vi "mupExpr Demo1.vi"() -> ()   [LabVIEW 2015]
uses:
  mupExpr/mupExpr.lvclass/mupExpr.ctl
  mupExpr/SetVarVal.vi
  mupLib/mupEval.vi
  mupLib/mupSetVarValue.vi
  mupLib/mupCheckError.vi
  mupLib/mupLibPath.vi
  <vilib>/Utility/error.llb/Error Cluster From Error Code.vi
  mupExpr/mupExpr.lvclass
panel:
  in  "Constants":cluster{"name":string, "value":dbl}[](array[cluster])=[{"name"="a", "value"=1.0}, {"name"="b", "value"=2.0}]
  out "error out":errorcluster
  out "XY Graph":cluster{dbl[], dbl[]}(graph)
  in  "Iterations":i32=1000
  out "Variable Names":string[](array[string])
  in  "Variable (x)":string="x"
  in  "Expression":string="a*x+b"
  in  "varValues (initial)":dbl[](array[numeric])=[0.0, 0.0, 0.0, 0.0, 0.0, 0.0] format="%#_13g"
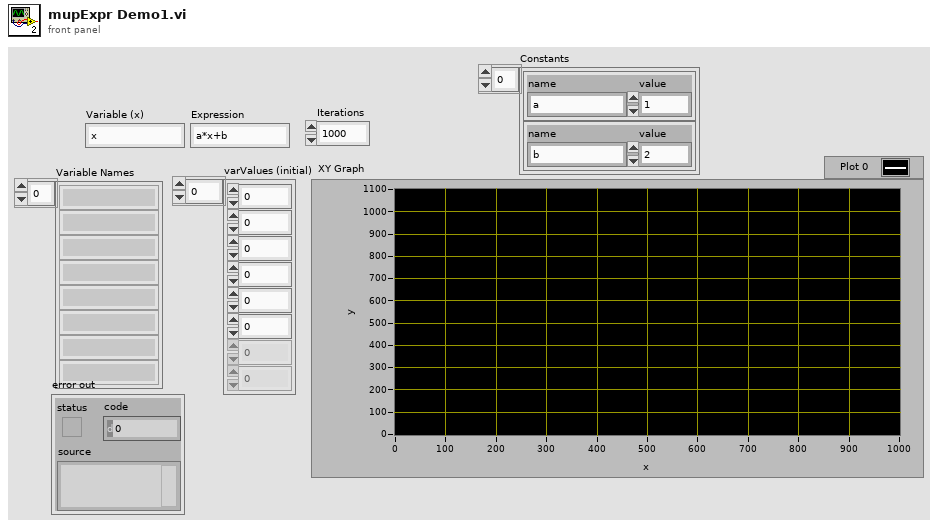
[diagram p1: front panel]
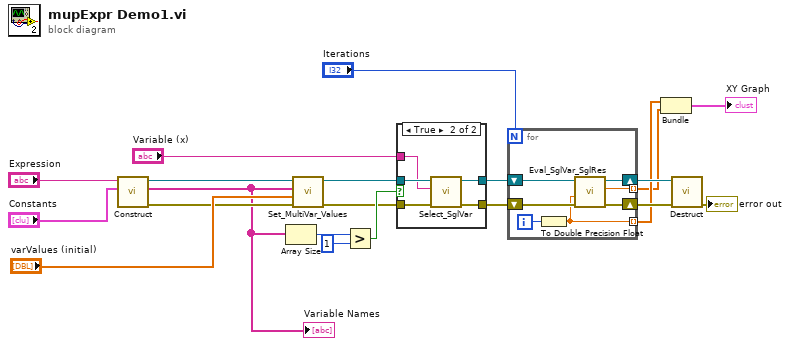
[diagram p0: block diagram]
diagram:
  n1 = call "Construct.vi"("Constants"="Constants", "Expression"="Expression") -> ("error out"=w19:errorcluster, "Variable Names"=w17:string[], "mupExpr out"=w21:refnum<data-value>)  [unwired: 7 in]
  "Variable Names" <- w17
  n2 = Array Size(array=w17) -> (size(s)=w16:i32)
  n3 = call "Set_MultiVar_Values.vi"("error in (no error)"=w19, "varValues"="varValues (initial)", "varNames"=w17, "mupExpr in"=w21) -> ("error out"=w12:errorcluster, "mupExpr out"=w13:refnum<data-value>)  [unwired: 6 in]
  n4 = Greater?(x=w16, y=1) -> (0:w14:bool)
  n5 = case shown="True" w14 {
    tunnel: w13 -> [w23 w28]
    tunnel: w12 -> [w22 w27]
    tunnel: [w22 w26] -> w8
    tunnel: [w23 w25] -> w10
    tunnel: "Variable (x)" -> [_ w24]
    frame False {
    }
    frame True {
      n6 = call "Select_SglVar.vi"("error in (no error)"=w27, "varName"=w24, "mupExpr in"=w28) -> ("error out"=w26:errorcluster, "mupExpr out"=w25:refnum<data-value>)  [unwired: 7 in]
    }
  }
  n7 = for {
    N: "Iterations" -> [_]
    shift-right: [w34] -> w9
    shift-left: w10 -> [w35]
    shift-right: [w32] -> w7
    shift-left: w8 -> [w33]
    tunnel: [w30] -> w4 mode=indexing
    tunnel: [w29] -> w5 mode=indexing
    i -> [w31]
    n8 = To Double Precision Float(number=w31) -> (double precision float=w29:dbl)
    n9 = call "Eval_SglVar_SglRes.vi"("error in (no error)"=w33, "varValue"=w29, "mupExpr in"=w35) -> ("error out"=w32:errorcluster, "Result"=w30:dbl, "mupExpr out"=w34:refnum<data-value>)  [unwired: 6 in]
  }
  n10 = Bundle(w5, w4) -> (→"XY Graph":cluster{dbl[], dbl[]})  [unwired: 1 in]
  n11 = call "Destruct.vi"("error in (no error)"=w7, "mupExpr in"=w9) -> ("error out"=→"error out":errorcluster)  [unwired: 9 in]
